vi "ModBus_RW_HoldingReg.vi"(0 "VISA Refnum in":refnum<visa-resource-name>, 1 "Func":u8, 2 "milliseconds to wait":u32=40, 3 "Num/ of sensor":i32, 5 "StartAdr":u16, 9 "Qanity":u16, 11 "error in (no error)":errorcluster, 12 "Data":string) -> (4 "VISA Refnum out":refnum<visa-resource-name>, 6 "read byte array":u8[](array[numeric]), 8 "read buffer":string, 13 "return count":u32, 14 "String w/o CRC":string, 15 "error out":errorcluster)   [LabVIEW 2018]
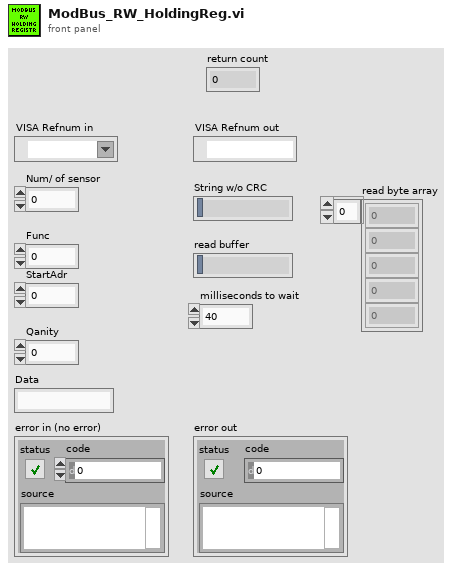
[diagram p1: front panel]
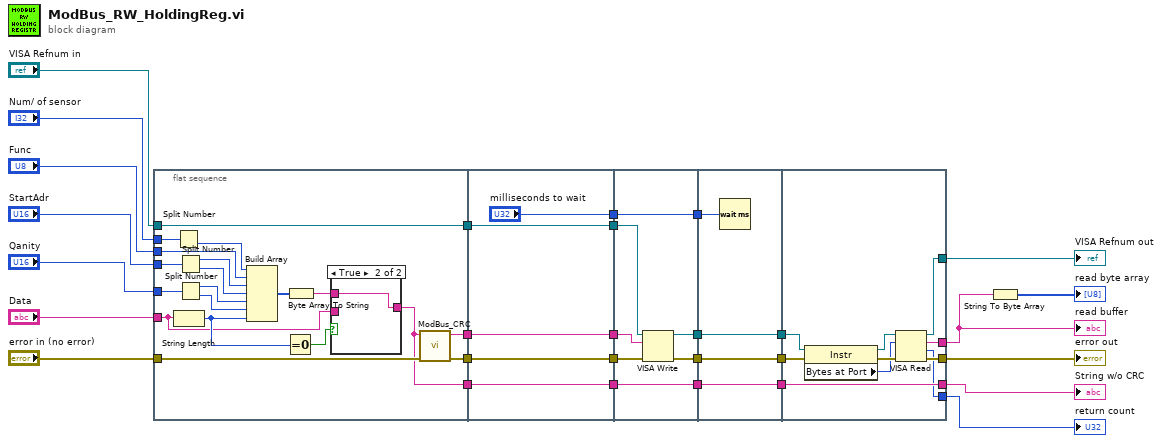
[diagram p0: block diagram]
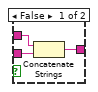
[diagram p2: hidden frame]
diagram:
  n1 = flat-sequence {
    tunnel: [w40] -> w29
    tunnel: "VISA Refnum in" -> [w40]
    tunnel: [w39] -> w28
    tunnel: "error in (no error)" -> [w38]
    tunnel: [w32] -> w27
    tunnel: "Num/ of sensor" -> [w37]
    tunnel: "Func" -> [w36]
    tunnel: "StartAdr" -> [w35]
    tunnel: "Qanity" -> [w34]
    tunnel: "Data" -> [w33]
    tunnel: [w31] -> w6
    tunnel: w29 -> [w57]
    tunnel: [w57] -> w26
    tunnel: w28 -> [w56]
    tunnel: [w56] -> w25
    tunnel: w27 -> [w55]
    tunnel: [w55] -> w24
    tunnel: ["milliseconds to wait"] -> w23
    tunnel: w6 -> [w53]
    tunnel: [w53] -> w5
    tunnel: w26 -> [w61]
    tunnel: w25 -> [w62]
    tunnel: w24 -> [w59]
    tunnel: [w64] -> w22
    tunnel: [w63] -> w21
    tunnel: w23 -> [w60]
    tunnel: [w60] -> w20
    tunnel: w5 -> [w58]
    tunnel: [w58] -> w4
    tunnel: w22 -> [w68]
    tunnel: [w68] -> w19
    tunnel: w21 -> [w67]
    tunnel: [w67] -> w18
    tunnel: w20 -> [w66]
    tunnel: w4 -> [w65]
    tunnel: [w65] -> w3
    tunnel: w19 -> [w76]
    tunnel: w18 -> [w77]
    tunnel: [w74] -> w16
    tunnel: [w70] -> w17
    tunnel: [w72] -> w8
    tunnel: w3 -> [w71]
    tunnel: [w71] -> w2
    tunnel: [w69] -> w1
    frame #0 {
      n2 = Split Number(x=w37) -> (lo(x)=w30:u16)  [unwired: 1 out]
      n3 = String Length(string=w33) -> (length=w41:i32)
      n4 = Split Number(x=w35) -> (hi(x)=w46:u8, lo(x)=w47:u8)
      n5 = Split Number(x=w34) -> (hi(x)=w43:u8, lo(x)=w42:u8)
      n6 = Build Array(w30, w36, w46, w47, w43, w42, w41) -> (w48:i32[])
      n7 = Equal To 0?(x=w41) -> (x = 0?=w44:bool)
      n8 = Byte Array To String(unsigned byte array=w48) -> (string=w45:string)
      n9 = case shown="True" w44 {
        tunnel: w45 -> [w51 w52]
        tunnel: [w50 w52] -> w31
        tunnel: w33 -> [w49 _]
        frame False {
          n10 = Concatenate Strings(w51, w49) -> (w50:string)
        }
        frame True {
        }
      }
      n11 = call "ModBus_CRC.vi"("error in (no error)"=w38, "string in"=w31) -> ("error out"=w39:errorcluster, "String + CRC"=w32:string)  [unwired: 8 in]
    }
    frame #1 {
    }
    frame #2 {
      n12 = VISA Write(VISA resource name=w61, write buffer=w59, error in (no error)=w62) -> (VISA resource name out=w63:refnum<visa-resource-name>, error out=w64:errorcluster)  [unwired: 1 out]
    }
    frame #3 {
      n13 = Wait (ms)(milliseconds to wait=w66) -> ()  [unwired: 1 out]
    }
    frame #4 {
      n14 = property class="Instr"(reference=w77, error in=w76) -> (reference out=w78:refnum<visa-resource-name>, error out=w75:errorcluster, "Bytes at Port"=w73:u32)
      n15 = VISA Read(VISA resource name=w78, byte count=w73, error in (no error)=w75) -> (VISA resource name out=w74:refnum<visa-resource-name>, read buffer=w72:string, return count=w69:u32, error out=w70:errorcluster)
    }
  }
  n16 = String To Byte Array(string=w8) -> (unsigned byte array=→"read byte array":u8[])
  "read buffer" <- w8
  "error out" <- w17
  "VISA Refnum out" <- w16
  "String w/o CRC" <- w2
  "return count" <- w1
